vi "Actor Core.vi"(8 "error in":errorcluster, 11 "AsmTestMachine in":refnum<class "AsmTestMachine.lvclass">) -> (0 "error out":errorcluster, 3 "Actor out":refnum<class "Actor.lvclass">)   [LabVIEW 2021, in "AsmTestMachine.lvlib" / "AsmTestMachine.lvclass"]
doc: "(<B>Filename</B>: Actor Framework.lvlib:Actor.lvclass:Actor Core.vi)\n\nReceives messages to the actor, reacts to them, and initiates any error handling that may shut the actor down.\n\nDescendant classes may override this VI to append parallel tasks for the actor to complete while it handles messages. Overrides use the Call Parent Class Method node."
uses:
  AsmTestMachine.lvclass
  C:/Program Files (x86)/National Instruments/LabVIEW 2021/vi.lib/ActorFramework/Actor/Actor.lvclass
  <vilib>/ActorFramework/Actor/Actor.lvclass
  Source/ActorStateMachine/ActorStateMachine/_ASM.State.ctl
  <vilib>/ActorFramework/Actor/Actor.lvclass/Actor.ctl
  <vilib>/ActorFramework/Message Enqueuer/Message Enqueuer.lvclass/Message Enqueuer.ctl
  AsmTestMachine.lvclass/AsmTestMachine.ctl
  <vilib>/ActorFramework/Message Enqueuer/Init from Existing Queue.vi
  <vilib>/ActorFramework/Message Enqueuer/Enqueue.vi
  Source/ActorStateMachine/ActorStateMachine Messages/ASM.Event.Quit Msg/ASM.Event.Quit Msg.lvclass
  C:/Program Files (x86)/National Instruments/LabVIEW 2021/vi.lib/ActorFramework/Message/Message.lvclass
  <vilib>/ActorFramework/Message Priority Queue/Priority Enqueue.vi
  <vilib>/ActorFramework/Message Enqueuer/Message Enqueuer.lvclass
  Source/ActorStateMachine/ActorStateMachine/ActorStateMachine.lvclass
  D:/_uliarczj/_sandbox/SWTest/Utilities/LabVIEW/ActorStateMachine/Source/ActorStateMachine/ActorStateMachine/ActorStateMachine.lvclass
  D:/_uliarczj/_sandbox/SWTest/Utilities/LabVIEW/ActorStateMachine/Test/AsmTestMachine/AsmTestMachine/AsmTestMachine.lvclass
panel:
  out "LedRunningIndicator":bool
  out "StateLog":string
  out "CurrentState":T1
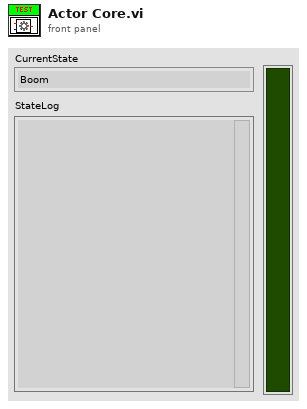
[diagram p1: front panel]
types:
  T1 = typedef "ActorStateMachine.lvlib/ActorStateMachine.lvclass/_ASM.State.ctl" = enum16{"Boom", "Pre-Init", "Init", "Post-Init", "Pre-Reset", "Reset", "Post-Reset", "Pre-Config", "Config", "Post-Config", "Pre-Ready", "Ready", "Post-Ready", "Pre-Running", "Running", "Next", "Post-Running", "Break", "Fail", "Crash", "Shutdown", "Doom"}
  T2 = cluster{"Stop":refnum<user-event>, "UpdateState":refnum<user-event>, "UpdateCustomMessage":refnum<user-event>}
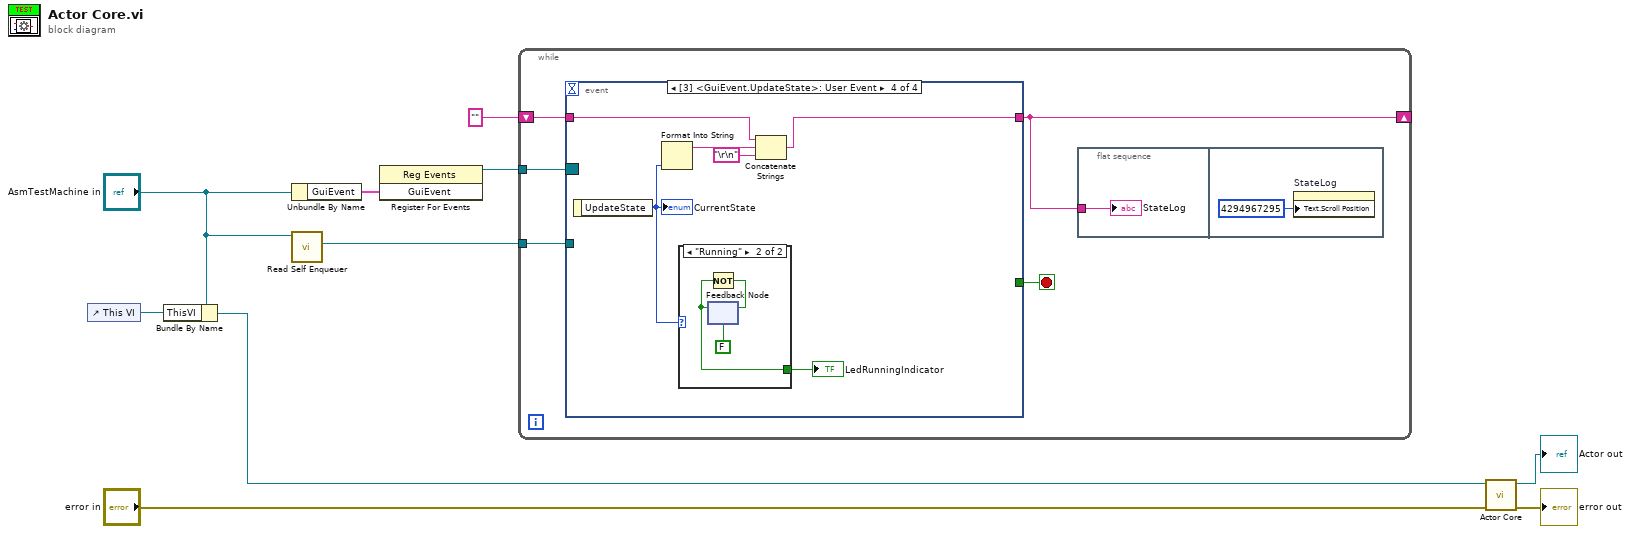
[diagram p0: block diagram]
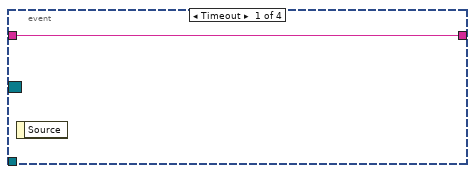
[diagram p2: hidden frame]
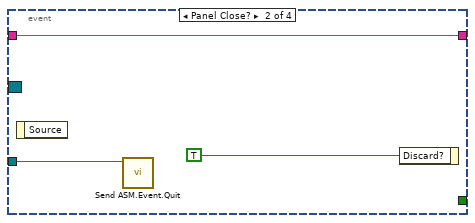
[diagram p3: hidden frame]
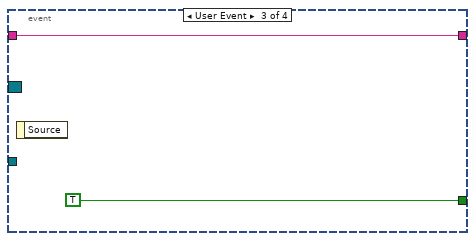
[diagram p4: hidden frame]
diagram:
  n1 = control-ref of="This VI"() -> (w7:refnum<vi>)
  n2 = Bundle By Name(cluster="AsmTestMachine in", "ThisVI"=w7) -> (w1:refnum<class "AsmTestMachine.lvclass">)
  n3 = Unbundle By Name("AsmTestMachine in") -> ("GuiEvent"=w6:T2)
  n4 = call <vilib>:"Read Self Enqueuer.vi"("Actor"="AsmTestMachine in") -> ("Self Enqueuer"=w3:refnum<class "Message Enqueuer.lvclass">)  [unwired: 10 in]
  n5 = register-events(w6) -> (reference out=w5:refnum<event-registration>)  [unwired: 2 in, 1 out]
  n6 = while {
    tunnel: w5 -> [w15]
    tunnel: w3 -> [w14]
    shift-right: [w11] -> _
    shift-left: "" -> [w12]
    stop <- w13 stop-if-true
    n7 = event shown="[3] <GuiEvent.UpdateState>: User Event" {
      selector: w15 -> [_ _ _ _]
      dyn-events: _ -> [_ _ _ _]
      timeout: _ -> [_ _ _ _]
      tunnel: w14 -> [_ w20 _ _]
      tunnel: [_ _ TRUE _] -> w13
      tunnel: [w18 w19 w22 w28] -> w11
      tunnel: w12 -> [w18 w19 w22 w27]
      event Timeout {
        n8 = event-data() -> ()  [unwired: 1 in, 1 out]
      }
      event Panel Close? {
        n9 = event-data() -> ()  [unwired: 1 in, 1 out]
        n10 = call "Send ASM.Event.Quit.vi"("Message Enqueuer"=w20) -> ()  [unwired: 9 in, 2 out]
        n11 = event-data("Discard?"=TRUE) -> ()  [unwired: 1 in, 1 out]
      }
      event User Event {
        n12 = event-data() -> ()  [unwired: 1 in, 1 out]
      }
      event User Event {
        n13 = event-data() -> ("UpdateState"=w25:T1)  [unwired: 1 in]
        "CurrentState" <- w25
        n14 = Format Into String(w25) -> (resulting string=w29:string)  [unwired: 3 in, 1 out]
        n15 = case shown="\"Running\"" w25 {
          tunnel: [_ w30] -> w24
          frame "Boom", Default {
          }
          frame "Running" {
            n16 = feedback #1(FALSE) -> (w30:bool)
            n17 = Not(x=w30) -> (.not. x?=w31:bool)
            n18 = feedback-in #1(w31) -> ()
          }
        }
        "LedRunningIndicator" <- w24
        n19 = Concatenate Strings(w27, w29, "\r\n") -> (w28:string)
      }
    }
    n20 = flat-sequence {
      tunnel: w11 -> [w16]
      frame #0 {
        "StateLog" <- w16
      }
      frame #1 {
        n21 = property on="StateLog" class="Str"("Text.Scroll Position"=u32 4294967295) -> ()  [unwired: 2 in, 2 out]
      }
    }
  }
  n22 = call-parent "Actor Core.vi"("error in"="error in", "Actor in"=w1) -> ("error out"=→"error out":errorcluster, "Actor out"=→"Actor out":refnum<class "Actor.lvclass">)  [unwired: 8 in]
